vi "SystemFlush.vi"(0 "VISA IN":refnum<visa-resource-name>, 5 "error in":errorcluster) -> (14 "VISA Out":refnum<visa-resource-name>, 19 "error out":errorcluster)   [LabVIEW 2018, in "PNA-X.lvlib"]
uses:
  PNA-X.lvlib
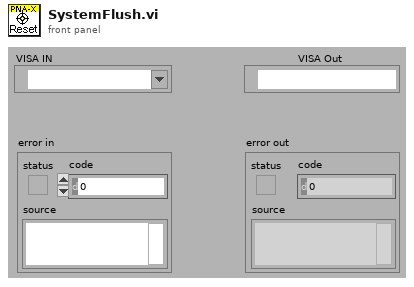
[diagram p1: front panel]
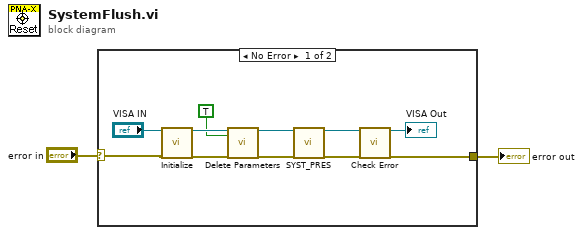
[diagram p0: block diagram]
diagram:
  n1 = case shown="No Error" "error in" {
    selector: "error in" -> [w11 w15]
    tunnel: [w13 w14] -> w2
    frame No Error {
      n2 = call "Initialize.vi"("VISA IN"="VISA IN", "error in"=w11) -> ("VISA Out"=w9:refnum<visa-resource-name>, "error out"=w10:errorcluster)  [unwired: 15 in, 1 out]
      n3 = call "Delete Parameters .vi"("VISA IN"=w9, "Delete All?"=TRUE, "error in"=w10) -> ("VISA Out"=w6:refnum<visa-resource-name>, "error out"=w3:errorcluster)  [unwired: 15 in]
      n4 = call "SYST_PRES.vi"("VISA IN"=w6, "error in"=w3) -> ("VISA Out"=w5:refnum<visa-resource-name>, "error out"=w4:errorcluster)  [unwired: 16 in]
      n5 = call "Check Error.vi"("VISA Resource Name"=w5, "error in (no error)"=w4) -> ("dup VISA session"=→"VISA Out":refnum<visa-resource-name>, "error out"=w13:errorcluster)  [unwired: 16 in]
    }
    frame Error {
      n6 = call <vilib>:"Simple Error Handler.vi"("error in (no error)"=w15) -> ("error out"=w14:errorcluster)  [unwired: 4 in, 4 out]
    }
  }
  "error out" <- w2
